vi "Generate Test Case.vi"(8 "error in (no error)":errorcluster, 9 "Directory":path, 10 "Name":string, 11 "Process Generator In":refnum<class "Process Generator.lvclass">) -> (0 "error out":errorcluster, 3 "Process Generator Out":refnum<class "Process Generator.lvclass">)   [LabVIEW 2020, in "Process Generator.lvclass"]
uses:
  Process Generator.lvclass
  Process Generator.lvclass/Process Generator.ctl
  <vilib>/Utility/traverseref.llb/TRef TravTarget.ctl
  <vilib>/Utility/traverseref.llb/VI Scripting - Traverse.lvlib
  <vilib>/Asteme/LUnit/Test Case.lvclass
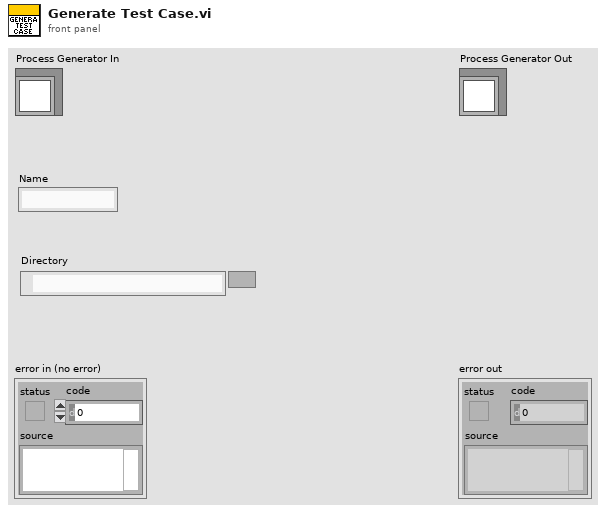
[diagram p1: front panel]
types:
  T1 = typedef "TRef TravTarget.ctl" = enum16{"FP", "BD", "Other"}
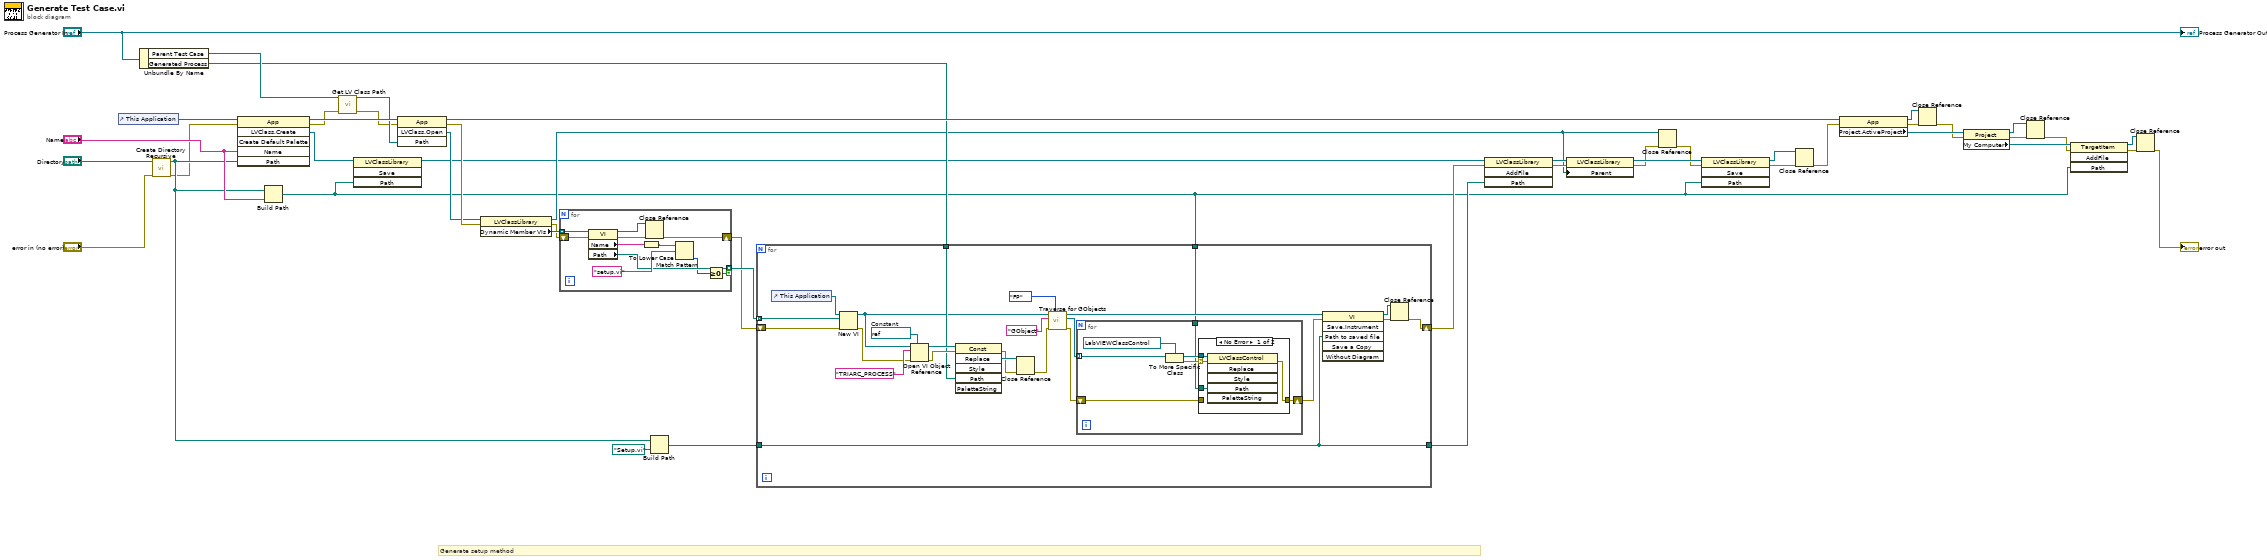
[diagram p0: block diagram]
diagram:
  # "Generate setup method"
  n1 = control-ref of="This Application"() -> (w13:refnum<vi>)
  n2 = Unbundle By Name("Process Generator In") -> ("Parent Test Case"=w46:refnum<class "Test Case.lvclass">, "Generated Process"=w20:path)
  n3 = call <vilib>:"Create Directory Recursive.vi"("error in (no error)"="error in (no error)", "directory"="Directory") -> ("error out"=w14:errorcluster, "directory copy"=w18:path)  [unwired: 3 in, 1 out]
  n4 = invoke class="App" method="LVClass.Create"(reference=w13, error in=w14, "Name"="Name", "Path"=w18) -> (reference out=w45:refnum<vi>, error out=w33:errorcluster, "LVClass.Create"=w3:refnum<vi>)  [unwired: 2 in, 3 out]
  n5 = Build Path(base path=w18, name or relative path="Name") -> (appended path=w1:path)
  n6 = call <vilib>:"Get LV Class Path.vi"("error in (no error)"=w33, "object"=w46) -> ("error out"=w32:errorcluster, "class path"=w44:path)  [unwired: 8 in]
  n7 = invoke class="LVClassLibrary" method="Save"(reference=w3, "Path"=w1) -> (reference out=w2:refnum<vi>)  [unwired: 2 in, 3 out]
  n8 = invoke class="App" method="LVClass.Open"(reference=w45, error in=w32, "Path"=w44) -> (reference out=w43:refnum<vi>, error out=w11:errorcluster, "LVClass.Open"=w6:refnum<vi>)  [unwired: 1 in, 1 out]
  n9 = property class="LVClassLibrary"(reference=w6, error in=w11) -> (reference out=w4:refnum<vi>, error out=w21:errorcluster, "Dynamic Member VIs"=w24:refnum<vi>[])
  n10 = for {
    tunnel: w24 -> [w58] mode=indexing
    shift-right: [w51] -> w22
    shift-left: w21 -> [w54]
    tunnel: [w52] -> w23 mode=indexing if=w49
    n11 = property class="VI"(reference=w58, error in=w54) -> (reference out=w50:refnum<vi>, error out=w53:errorcluster, "Name"=w57:string, "Path"=w52:path)
    n12 = To Lower Case(string=w57) -> (all lower case string=w56:string)
    n13 = Close Reference(reference=w50, error in (no error)=w53) -> (error out=w51:errorcluster)
    n14 = Match Pattern(string=w56, regular expression="setup.vi" ("y")) -> (offset past match=w48:i32)  [unwired: 1 in, 3 out]
    n15 = Greater Or Equal To 0?(x=w48) -> (x >= 0?=w49:bool)
  }
  n16 = Build Path(base path=w18, name or relative path=path "Setup.vi") -> (appended path=w16:path)
  n17 = for {
    tunnel: w23 -> [w82] mode=indexing
    shift-right: [w71] -> w19
    shift-left: w22 -> [w81]
    tunnel: w20 -> [w75]
    tunnel: w16 -> [w69]
    tunnel: [w69] -> w15
    tunnel: w1 -> [w62]
    w79 = refnum<vi> refnum  # Constant
    n18 = control-ref of="This Application"() -> (w59:refnum<vi>)
    n19 = New VI(8:w81, 10:w82, 11:w59) -> (0:w78:errorcluster, 3:w68:refnum<vi>)  [unwired: 4 in]
    n20 = Open VI Object Reference(7:w79, 8:w78, 10:"TRIARC_PROCESS" ("name/order"), 11:w68) -> (0:w76:errorcluster, 3:w77:refnum<vi>)
    n21 = invoke on="Invoke Node" class="Const" method="Replace"(reference=w77, error in=w76, "Path"=w75) -> (error out=w73:errorcluster, "Replace"=w74:refnum<vi>)  [unwired: 3 in, 4 out]
    n22 = Close Reference(reference=w74, error in (no error)=w73) -> (error out=w64:errorcluster)
    n23 = call <vilib>:"Traverse for GObjects.vi"("Traverse Target"=TRef_TravTarget."FP", "error in (no error)"=w64, "Class Name"="GObject", "VI Refnum"=w68) -> ("error out"=w60:errorcluster, "References"=w63:refnum<vi>[], "dup VI Refnum"=w67:refnum<vi>)  [unwired: 4 in, 1 out]
    n24 = for {
      tunnel: w63 -> [w89] mode=indexing
      tunnel: w62 -> [w85]
      shift-right: [w84] -> w61
      shift-left: w60 -> [w83]
      n25 = To More Specific Class(target class=refnum<vi> refnum ("reference out"), reference=w89) -> (specific class reference=w86:refnum<vi>, error out=w87:errorcluster)  [unwired: 1 in]
      n26 = case shown="No Error" w87 {
        selector: w87 -> [w93 _]
        tunnel: w86 -> [w92 _]
        tunnel: w85 -> [w91 _]
        tunnel: [w90 w94] -> w84
        tunnel: w83 -> [_ w94]
        frame No Error {
          n27 = invoke on="Invoke Node" class="LVClassControl" method="Replace"(reference=w92, error in=w93, "Path"=w91) -> (error out=w90:errorcluster)  [unwired: 3 in, 5 out]
        }
        frame Error {
        }
      }
    }
    n28 = invoke on="Invoke Node" class="VI" method="Save.Instrument"(reference=w67, error in=w61, "Path to saved file"=w69) -> (reference out=w70:refnum<vi>, error out=w72:errorcluster)  [unwired: 3 in, 4 out]
    n29 = Close Reference(reference=w70, error in (no error)=w72) -> (error out=w71:errorcluster)
  }
  n30 = invoke class="LVClassLibrary" method="AddFile"(reference=w2, error in=w19, "Path"=w15) -> (reference out=w10:refnum<vi>, error out=w8:errorcluster)  [unwired: 1 in, 2 out]
  n31 = property class="LVClassLibrary"(reference=w10, error in=w8, "Parent"=w4) -> (reference out=w9:refnum<vi>, error out=w7:errorcluster)
  n32 = Close Reference(reference=w4, error in (no error)=w7) -> (error out=w5:errorcluster)
  n33 = invoke class="LVClassLibrary" method="Save"(reference=w9, error in=w5, "Path"=w1) -> (reference out=w12:refnum<vi>, error out=w39:errorcluster)  [unwired: 1 in, 2 out]
  n34 = Close Reference(reference=w12, error in (no error)=w39) -> (error out=w37:errorcluster)
  n35 = property class="App"(reference=w43, error in=w37) -> (reference out=w30:refnum<vi>, error out=w41:errorcluster, "Project.ActiveProject"=w42:refnum<vi>)
  n36 = Close Reference(reference=w30, error in (no error)=w41) -> (error out=w31:errorcluster)
  n37 = property class="Project"(reference=w42, error in=w31) -> (reference out=w28:refnum<vi>, error out=w36:errorcluster, "My Computer"=w40:refnum<vi>)
  n38 = Close Reference(reference=w28, error in (no error)=w36) -> (error out=w29:errorcluster)
  n39 = invoke class="TargetItem" method="AddFile"(reference=w40, error in=w29, "Path"=w1) -> (reference out=w26:refnum<vi>, error out=w35:errorcluster)  [unwired: 1 in, 2 out]
  n40 = Close Reference(reference=w26, error in (no error)=w35) -> (error out=→"error out":errorcluster)
  "Process Generator Out" <- "Process Generator In"
